vi "Formula Node.vi"() -> ()   [LabVIEW 2018]
panel:
  out "Waveform Graph":dbl[](graph)
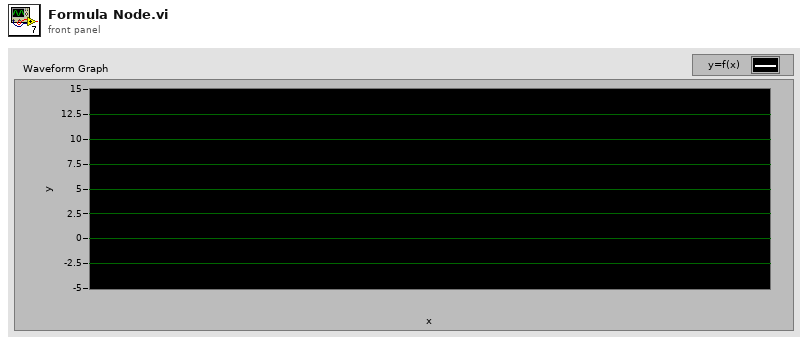
[diagram p1: front panel]
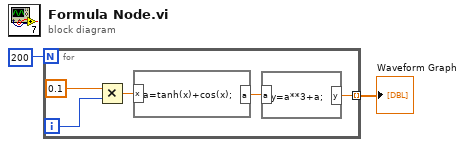
[diagram p0: block diagram]
diagram:
  n1 = for {
    N: 200 -> [_]
    tunnel: [w5] -> w1 mode=indexing
    i -> [w3]
    n2 = Multiply(x=0.1, y=w3) -> (x*y=w7:dbl)
    n3 = formula code="a=tanh(x)+cos(x);"("x"=w7) -> ("a"=w6:dbl)
    n4 = formula code="y=a**3+a;"("a"=w6) -> ("y"=w5:dbl)
  }
  "Waveform Graph" <- w1
